vi "ziExample-HF2-RTK-PI.vi"() -> ()   [LabVIEW 2009]
doc: "This is an example for a Zurich Instruments HF2 instrument with RTK option installed. \nThis VI works together with a program for the real-time processor to implement two PI (Proportional-Integral) controllers. The controllers themselves run on the real-time processor. This VI communicates with the real-time processor to configure the controllers.\nThe program for the real-time processor is implemented in the file Main.c."
uses:
  <instrlib>/Zurich Instruments LabOne/Zurich Instruments LabOne.lvlib
panel:
  in  "pid2_invert":bool
  in  "pid1_invert":bool
  in  "pid2_input_select2":enum16{"X", "Y", "R", "Theta"}(ring) caption="Signal"
  in  "pid1_input_select2":enum16{"X", "Y", "R", "Theta"}(ring) caption="Signal"
  in  "pid2_max":sgl=1.0 format="%+7.3f"
  in  "pid2_min":sgl=-1.0 caption="Range" format="%+7.3f"
  in  "pid1_max":sgl=1.0 format="%+7.3f"
  in  "pid1_min":sgl=-1.0 caption="Range" format="%+7.3f"
  in  "pid2_output_select":enum16{"Aux 1", "Aux 2", "Aux 3", "Aux 4"}(ring)=enum."Aux 2" caption="Output"
  in  "pid1_output_select":enum16{"Aux 1", "Aux 2", "Aux 3", "Aux 4"}(ring) caption="Output"
  in  "stop":bool
  out "pid2_error":dbl caption="Error" format="%_5p"
  out "pid1_error":dbl caption="Error" format="%_5p"
  in  "Port":u16=8005
  in  "Host":string="localhost"
  in  "pid2_enable":bool caption="demodOn0"
  in  "pid1_enable":bool
  in  "pid2_set_point":sgl caption="Set point" format="%+7.3f"
  in  "pid2_tc_slider":sgl(slide)=1.0 scale=0.001..10.0 scale format="%#_6p"
  in  "pid2_kp_slider":sgl(slide)=0.001 scale=0.001..1.0 scale format="%#_6p"
  in  "pid2_input_select1":T1(ring)=enum."Demod 2" caption="Demodulator"
  in  "pid1_set_point":sgl caption="Set point" format="%+7.3f"
  in  "pid1_tc_slider":sgl(slide)=1.0 scale=0.001..10.0 scale format="%#_6p"
  in  "pid1_kp_slider":sgl(slide)=0.001 scale=0.001..1.0 scale format="%#_6p"
  in  "pid1_input_select1":T1(ring) caption="Demodulator"
  # "Prop. gain"
  # "Time constant (s)"
  # "En"
  # "Inv"
  # "Tested Devices:\n- HF2LI\n\nRequires the RTK \noption"
  # "PID1"
  # "to"
  # "Prop. gain"
  # "Time constant (s)"
  # "En"
  # "Inv"
  # "PID2"
  # "to"
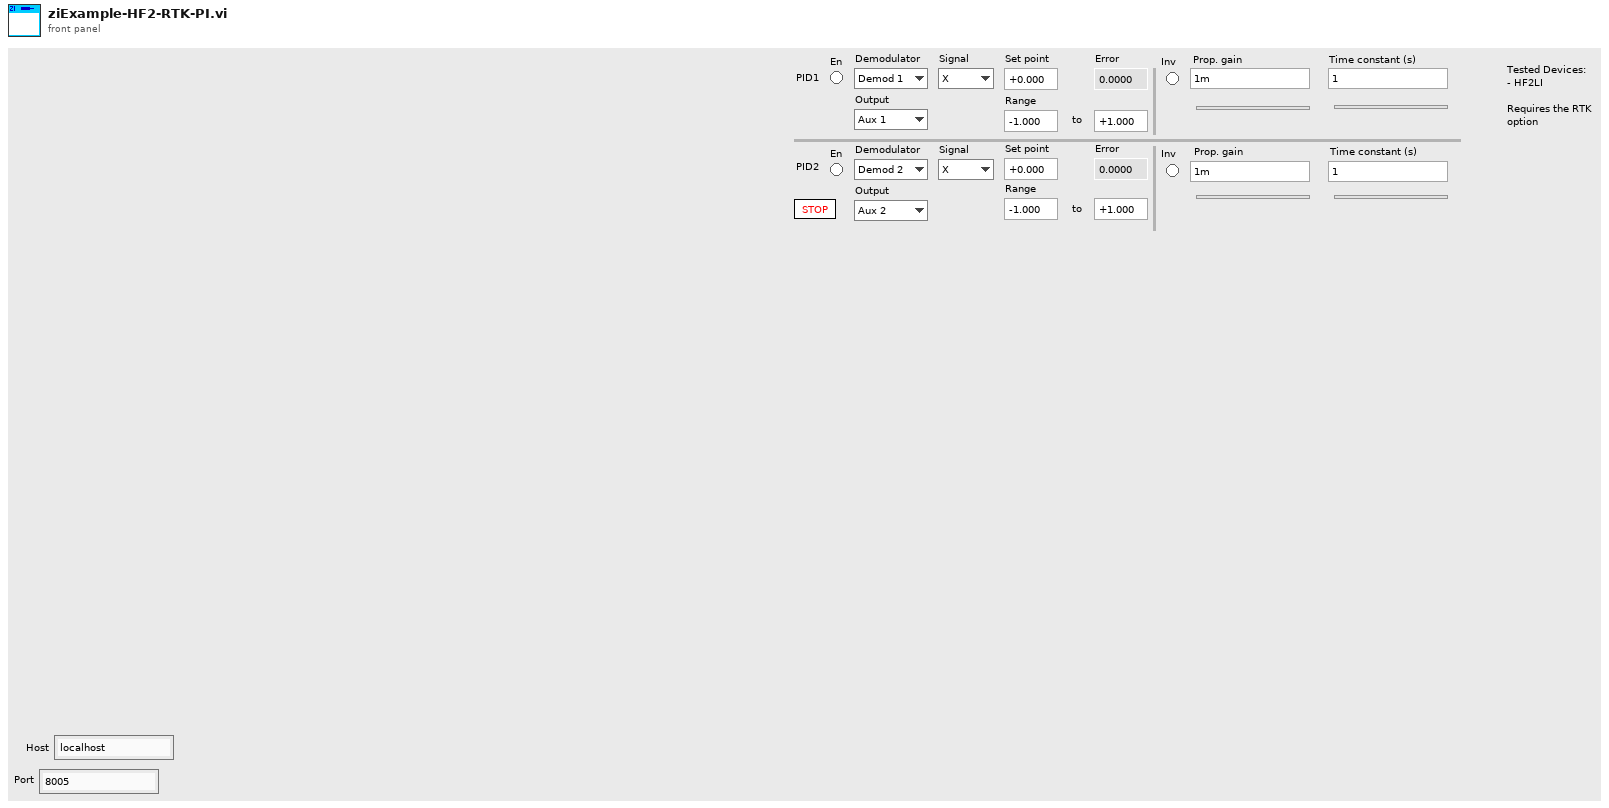
[diagram p1: front panel]
types:
  T1 = enum16{"Demod 1", "Demod 2", "Demod 3", "Demod 4", "Demod 5", "Demod 6", "Aux In 1", "Aux In 2"}
  T2 = typedef "Zurich Instruments LabOne.lvlib/ziTypeHandle.ctl" = cluster{"handleValid":bool, "Conn":u64, "Path Prefix":string, "Handle":u64, "Connected":bool, "Clockbase(s)":dbl}
  T3 = enum8{"Enabled", "Disabled", "Disabled and Grayed Out"}
  T4 = typedef "Zurich Instruments LabOne.lvlib/ziTypePollData.ctl" = cluster{"double":dbl, "Demod Sample":T5, "string":string, "Raw":u8[], "int":i32, "ScopeData":cluster{"wave":i16[], "dt (s)":dbl}, "DioInput":cluster{"Timestamp (ticks)":u64[], "Value":u32[]}, "AuxInput":cluster{"Timestamp (ticks)":u64[], "Val Ch0 (V)":dbl[], "Val Ch1 (V)":dbl[]}}
  T5 = typedef "Zurich Instruments LabOne.lvlib/ziTypeDemodSample.ctl" = cluster{"Channel":i32, "Timestamps (ticks)":u64[], "X (Vrms)":dbl[], "Y (Vrms)":dbl[], "Osc Phase (deg)":dbl[], "Freq (Hz)":dbl[], "DIO":u32[], "Aux In 0 (V)":dbl[], "Aux In 1 (V)":dbl[]}
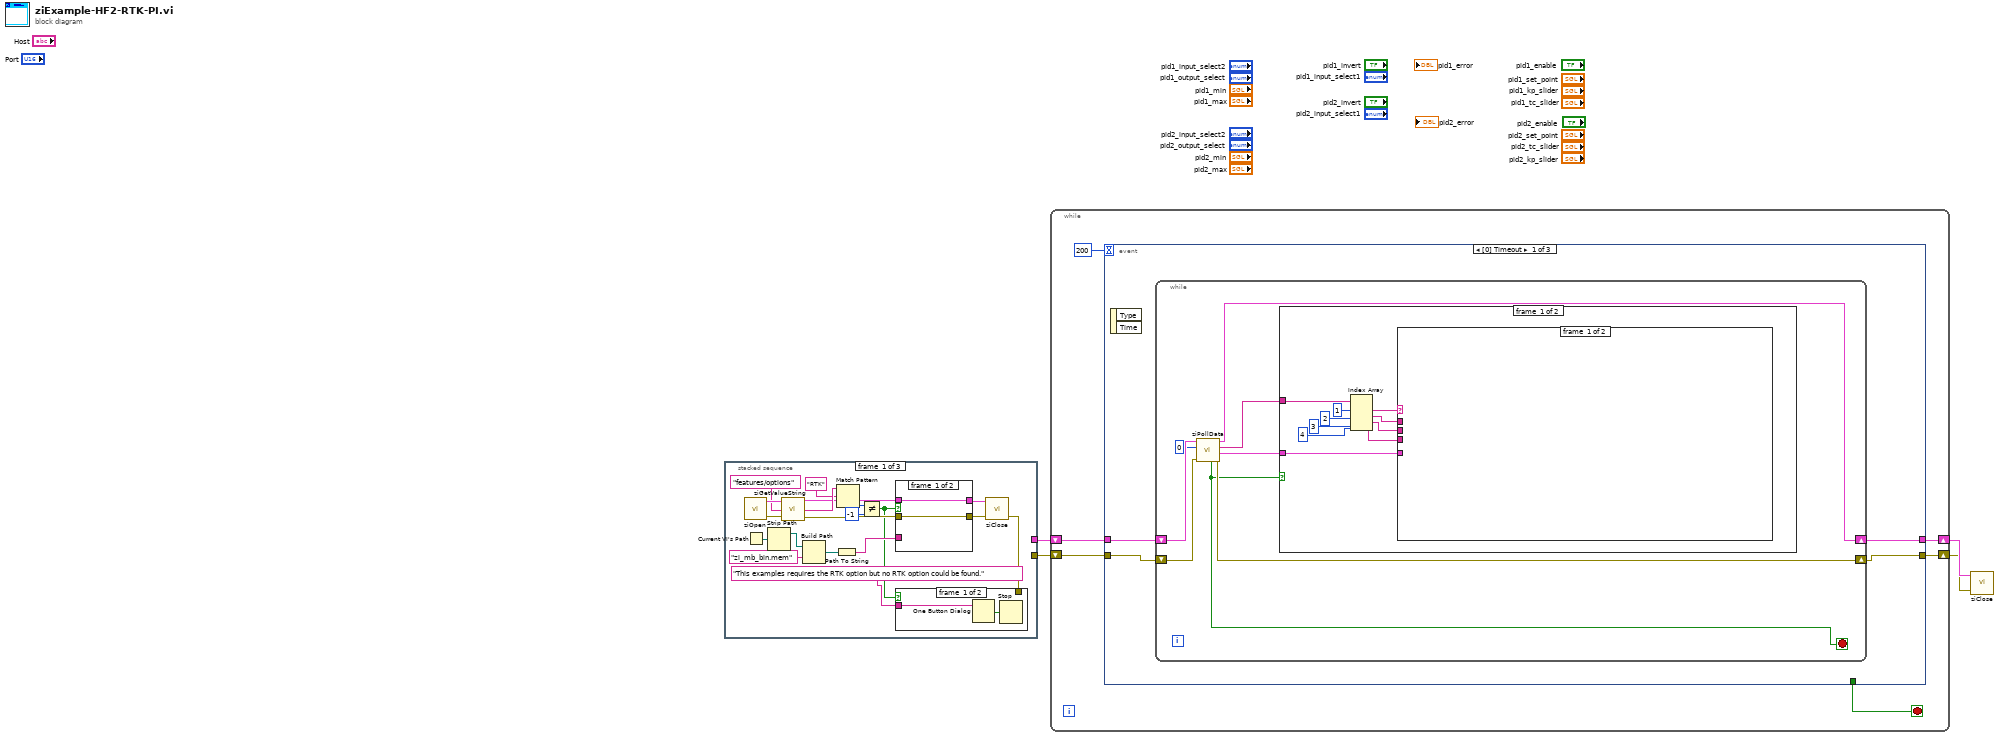
[diagram p0: block diagram]
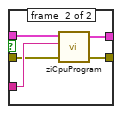
[diagram p3: hidden frame]
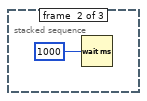
[diagram p4: hidden frame]
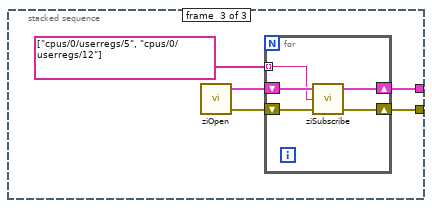
[diagram p5: hidden frame]
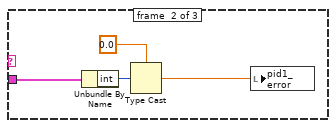
[diagram p9: hidden frame]
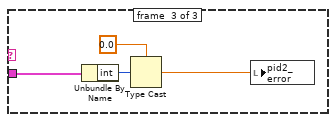
[diagram p10: hidden frame]
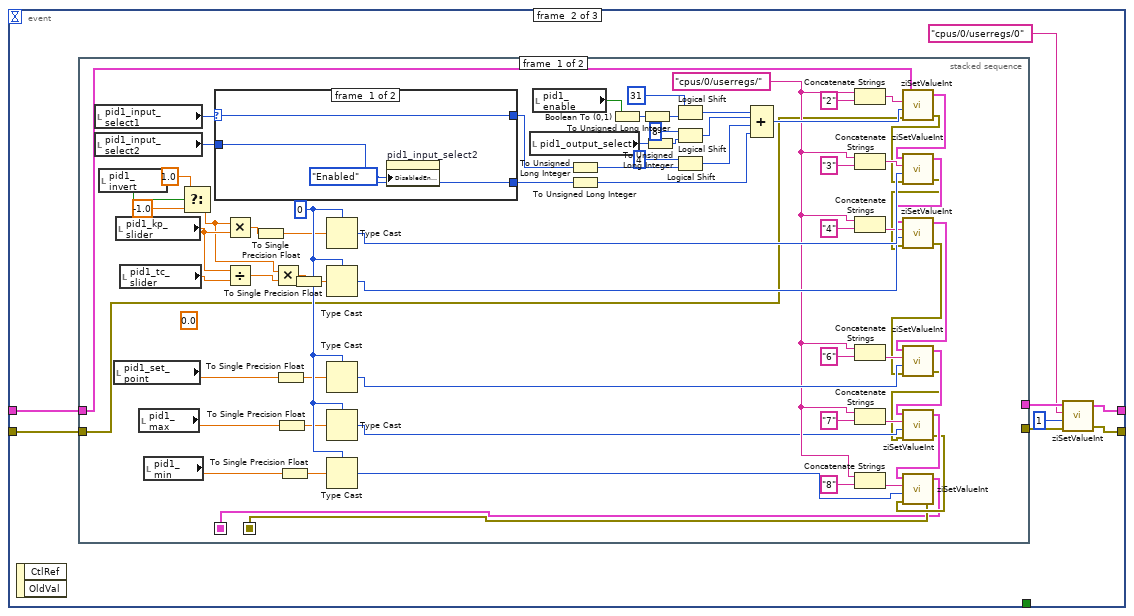
[diagram p12: hidden frame]
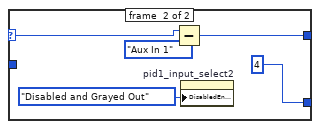
[diagram p13: hidden frame]
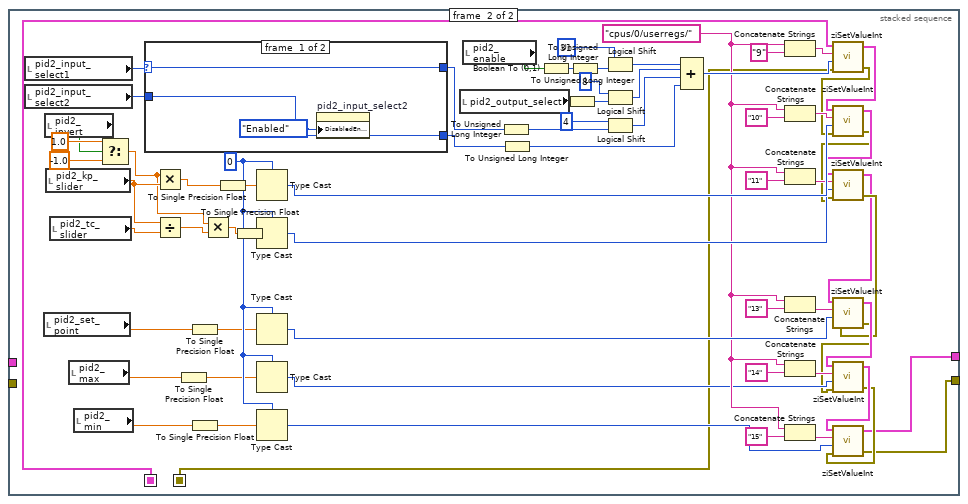
[diagram p14: hidden frame]
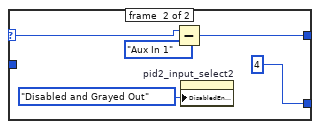
[diagram p15: hidden frame]
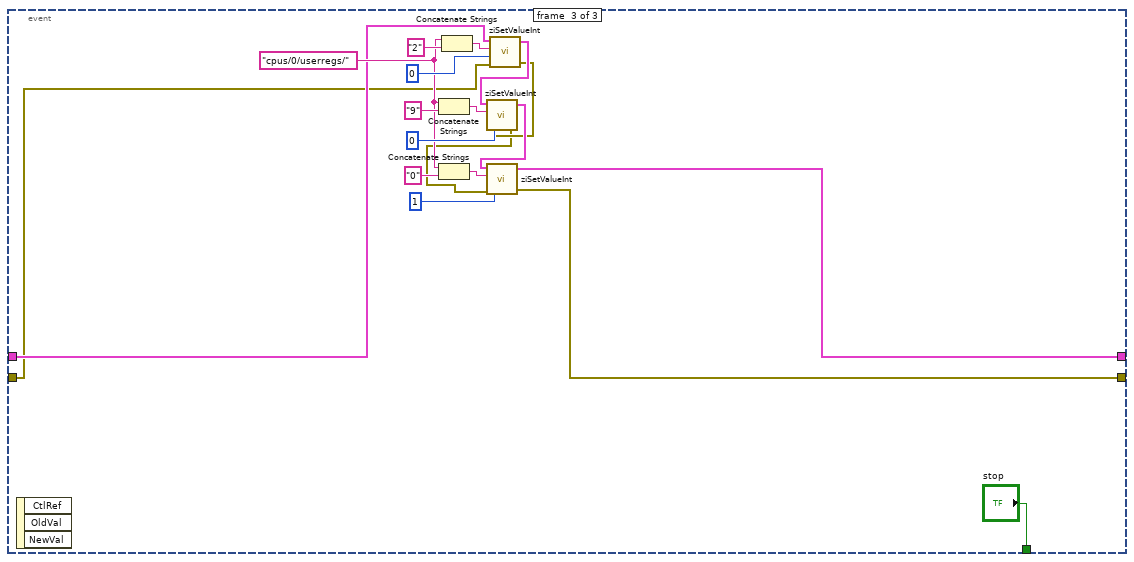
[diagram p16: hidden frame]
diagram:
  n1 = stacked-sequence {
    tunnel: [_ _ w37] -> w2
    tunnel: [_ _ w36] -> w1
    frame #0 {
      n2 = call <instrlib>:"ziOpen.vi"() -> ("Error Out"=w15:errorcluster, "HandleOut"=w16:T2)  [unwired: 4 in, 1 out]
      n3 = Current VI's Path() -> (path=w18:path)
      n4 = Strip Path(path=w18) -> (stripped path=w19:path)  [unwired: 1 out]
      n5 = call <instrlib>:"ziGetValueString.vi"("error in"=w15, "Path"="features/options", "Handle In"=w16) -> ("error out"=w9:errorcluster, "Value"=w13:string, "Handle Out"=w8:T2)
      n6 = Build Path(base path=w19, name or relative path="zi_mb_bin.mem") -> (appended path=w17:path)
      n7 = Path To String(path=w17) -> (string=w20:string)
      n8 = Match Pattern(string=w13, regular expression="RTK" ("Path")) -> (offset past match=w11:i32)  [unwired: 1 in, 3 out]
      n9 = Not Equal?(x=w11, y=-1) -> (x != y?=w7:bool)
      n10 = case shown="False" w7 {
        tunnel: [w26 w32] -> w22
        tunnel: [w27 w31] -> w21
        tunnel: w20 -> [_ w30]
        tunnel: w9 -> [w26 w29]
        tunnel: w8 -> [w27 w28]
        frame #0 {
        }
        frame #1 {
          n11 = call <instrlib>:"ziCpuProgram.vi"("error in"=w29, "Filename"=w30, "Handle In"=w28) -> ("error out"=w32:errorcluster, "Handle Out"=w31:T2)  [unwired: 2 in]
        }
      }
      n12 = call <instrlib>:"ziClose.vi"("Error In"=w22, "Handle In"=w21) -> ("Error Out"=w6:errorcluster)  [unwired: 3 out]
      n13 = case shown="False" w7 {
        tunnel: w6 -> [_ _]
        tunnel: "This examples requires the RTK option but no RTK option could be found." ("message") -> [w24 _]
        frame #0 {
          n14 = One Button Dialog(message=w24) -> (true=w25:bool)  [unwired: 1 in]
          n15 = Stop(stop? (T)=w25) -> ()
        }
        frame #1 {
        }
      }
    }
    frame #1 {
      n16 = Wait (ms)(milliseconds to wait=u32 1000) -> ()  [unwired: 1 out]
    }
    frame #2 {
      n17 = call <instrlib>:"ziOpen.vi"() -> ("Error Out"=w34:errorcluster, "HandleOut"=w35:T2)  [unwired: 4 in, 1 out]
      n18 = for {
        shift-right: [w41] -> w37
        shift-left: w35 -> [w43]
        shift-right: [w40] -> w36
        shift-left: w34 -> [w42]
        tunnel: string[] ["cpus/0/userregs/5", "cpus/0/userregs/12"] -> [w39] mode=indexing
        n19 = call <instrlib>:"ziSubscribe.vi"("error in"=w42, "Path ()"=w39, "Handle In"=w43) -> ("error out"=w40:errorcluster, "Handle Out"=w41:T2)  [unwired: 1 in]
      }
    }
  }
  n20 = while {
    shift-right: [w47] -> w4
    shift-left: w2 -> [w49]
    shift-right: [w46] -> w3
    shift-left: w1 -> [w48]
    stop <- w45 stop-if-true
    n21 = event shown="[0] Timeout" {
      selector: _ -> [_ _ _]
      dyn-events: _ -> [_ _ _]
      timeout: 200 -> [_ _ _]
      tunnel: w49 -> [w53 w96 w256]
      tunnel: w48 -> [w52 w95 w252]
      tunnel: [w51 w93 w255] -> w47
      tunnel: [w50 w94 w249] -> w46
      tunnel: [_ _ "stop"] -> w45
      event #0 {
        n22 = event-data() -> ()  [unwired: 3 out]
        n23 = while {
          shift-right: [w59] -> w51
          shift-left: w53 -> [w61]
          shift-right: [w58] -> w50
          shift-left: w52 -> [w60]
          stop <- w57 stop-if-true
          n24 = call <instrlib>:"ziPollData.vi"("Error In"=w60, "TimeOut ms (50)"=0, "Handle In"=w61) -> ("Error Out"=w58:errorcluster, "Data Out"=w55:T4, "PathArray"=w56:string[], "Handle Out"=w59:T2, "Timed Out"=w57:bool)  [unwired: 3 in, 1 out]
          n25 = case shown="False" w57 {
            tunnel: w56 -> [w71 _]
            tunnel: w55 -> [w66 _]
            frame #0 {
              n26 = Index Array(array=w71, index #1=1 ("index"), index #2=2 ("index"), index #3=3 ("index"), index #4=4 ("index")) -> (element #1=w69:string, element #2=w67:string, element #3=w64:string, element #4=w62:string)
              n27 = case shown="\"CPUS\"" w69 {
                tunnel: w67 -> [_ w75]
                tunnel: w66 -> [_ w73]
                tunnel: w64 -> [_ w74]
                tunnel: w62 -> [_ w72]
                frame #0 {
                }
                frame #1 {
                  n28 = case shown="\"0\"" w75 {
                    tunnel: w74 -> [_ w78]
                    tunnel: w73 -> [_ w77]
                    tunnel: w72 -> [_ w76]
                    frame #0 {
                    }
                    frame #1 {
                      n29 = case shown="\"USERREGS\"" w78 {
                        tunnel: w77 -> [_ w79]
                        tunnel: w76 -> [_ w80]
                        frame #0 {
                        }
                        frame #1 {
                          n30 = case shown="\"5\"" w80 {
                            tunnel: w79 -> [_ w84 w88]
                            frame #0 {
                            }
                            frame #1 {
                              n31 = Unbundle By Name(w84) -> ("int"=w83:i32)
                              n32 = Type Cast(type=sgl 0.0, x=w83) -> (*(type *) &x=w81:sgl)
                              n33 = local write "pid1_error"(w81) -> ()
                            }
                            frame #2 {
                              n34 = Unbundle By Name(w88) -> ("int"=w87:i32)
                              n35 = Type Cast(type=sgl 0.0, x=w87) -> (*(type *) &x=w85:sgl)
                              n36 = local write "pid2_error"(w85) -> ()
                            }
                          }
                        }
                      }
                    }
                  }
                }
              }
            }
            frame #1 {
            }
          }
        }
      }
      event #1 {
        n37 = event-data() -> ()  [unwired: 3 out]
        n38 = stacked-sequence {
          seq-local: [w115 _] -> [_ w193]
          seq-local: [w116 _] -> [_ w192]
          tunnel: w96 -> [w126 _]
          tunnel: w95 -> [w125 _]
          tunnel: [_ w195] -> w91
          tunnel: [_ w194] -> w92
          frame #0 {
            w136 = 0
            w129 = "cpus/0/userregs/"
            (unwired) sgl 0.0 ("number")
            n39 = local read "pid1_input_select1"() -> (w162:T1)
            n40 = local read "pid1_input_select2"() -> (w161:enum16{"X", "Y", "R", "Theta"})
            n41 = local read "pid1_invert"() -> (w106:bool)
            n42 = local read "pid1_set_point"() -> (w140:sgl)
            n43 = local read "pid1_kp_slider"() -> (w164:sgl)
            n44 = local read "pid1_tc_slider"() -> (w163:sgl)
            n45 = local read "pid1_max"() -> (w135:sgl)
            n46 = local read "pid1_min"() -> (w134:sgl)
            n47 = Select(t=1.0, s=w106, f=-1.0) -> (s? t:f=w102:dbl)
            n48 = case shown="\"Aux In 1\", \"Aux In 2\"" w162 {
              selector: w162 -> [w167 w172]
              tunnel: [w167 w170] -> w154
              tunnel: [w166 4] -> w153
              tunnel: w161 -> [w166 _]
              frame #0 {
                n49 = property on="pid1_input_select2" class="Enum (strict)"("DisabledEnum"=T3."Enabled" ("Disabled")) -> ()  [unwired: 2 in, 2 out]
              }
              frame #1 {
                n50 = Subtract(x=w172, y=T1."Aux In 1") -> (x-y=w170:u16)
                n51 = property on="pid1_input_select2" class="Enum (strict)"("DisabledEnum"=T3."Disabled and Grayed Out" ("Disabled")) -> ()  [unwired: 2 in, 2 out]
              }
            }
            n52 = Multiply(x=w102, y=w164) -> (x*y=w146:dbl)
            n53 = Divide(x=w164, y=w163) -> (x/y=w103:sgl)
            n54 = To Single Precision Float(number=w146) -> (single precision float=w101:sgl)
            n55 = Multiply(x=w102, y=w103) -> (x*y=w144:dbl)
            n56 = To Single Precision Float(number=w140) -> (single precision float=w99:sgl)
            n57 = To Single Precision Float(number=w135) -> (single precision float=w98:sgl)
            n58 = To Single Precision Float(number=w134) -> (single precision float=w97:sgl)
            n59 = To Single Precision Float(number=w144) -> (single precision float=w100:sgl)
            n60 = Type Cast(type=w136, x=w101) -> (*(type *) &x=w145:i32)
            n61 = Type Cast(type=w136, x=w100) -> (*(type *) &x=w141:i32)
            n62 = Type Cast(type=w136, x=w99) -> (*(type *) &x=w137:i32)
            n63 = Type Cast(type=w136, x=w98) -> (*(type *) &x=w127:i32)
            n64 = Type Cast(type=w136, x=w97) -> (*(type *) &x=w128:i32)
            n65 = local read "pid1_output_select"() -> (w149:enum16{"Aux 1", "Aux 2", "Aux 3", "Aux 4"})
            n66 = local read "pid1_enable"() -> (w160:bool)
            n67 = To Unsigned Long Integer(number=w154) -> (unsigned 32bit integer=w113:u32)
            n68 = To Unsigned Long Integer(number=w153) -> (unsigned 32bit integer=w110:u32)
            n69 = Boolean To (0,1)(Boolean=w160) -> (0, 1=w158:i16)
            n70 = To Unsigned Long Integer(number=w158) -> (unsigned 32bit integer=w114:u32)
            n71 = To Unsigned Long Integer(number=w149) -> (unsigned 32bit integer=w112:u32)
            n72 = Logical Shift(y=u32 31, x=w114) -> (x << y=w156:u32)
            n73 = Logical Shift(y=u32 8, x=w112) -> (x << y=w111:u32)
            n74 = Logical Shift(y=u32 4, x=w113) -> (x << y=w109:u32)
            n75 = Compound Arithmetic op=ADD(w156, w111, w109, w110) -> (w159:u32)
            n76 = Concatenate Strings(w129, "2" ("string")) -> (w152:string)
            n77 = Concatenate Strings(w129, "3" ("string")) -> (w148:string)
            n78 = Concatenate Strings(w129, "4" ("string")) -> (w143:string)
            n79 = Concatenate Strings(w129, "6" ("string")) -> (w139:string)
            n80 = Concatenate Strings(w129, "7" ("string")) -> (w132:string)
            n81 = Concatenate Strings(w129, "8" ("string")) -> (w131:string)
            n82 = call <instrlib>:"ziSetValueInt.vi"("Error in"=w125, "Value"=w159, "Path"=w152, "Handle in"=w126) -> ("Error out"=w120:errorcluster, "Handle out"=w124:T2)  [unwired: 1 in]
            n83 = call <instrlib>:"ziSetValueInt.vi"("Error in"=w120, "Value"=w145, "Path"=w148, "Handle in"=w124) -> ("Error out"=w119:errorcluster, "Handle out"=w123:T2)  [unwired: 1 in]
            n84 = call <instrlib>:"ziSetValueInt.vi"("Error in"=w119, "Value"=w141, "Path"=w143, "Handle in"=w123) -> ("Error out"=w108:errorcluster, "Handle out"=w107:T2)  [unwired: 1 in]
            n85 = call <instrlib>:"ziSetValueInt.vi"("Error in"=w108, "Value"=w137, "Path"=w139, "Handle in"=w107) -> ("Error out"=w118:errorcluster, "Handle out"=w122:T2)  [unwired: 1 in]
            n86 = call <instrlib>:"ziSetValueInt.vi"("Error in"=w118, "Value"=w127, "Path"=w132, "Handle in"=w122) -> ("Error out"=w117:errorcluster, "Handle out"=w121:T2)  [unwired: 1 in]
            n87 = call <instrlib>:"ziSetValueInt.vi"("Error in"=w117, "Value"=w128, "Path"=w131, "Handle in"=w121) -> ("Error out"=w116:errorcluster, "Handle out"=w115:T2)  [unwired: 1 in]
          }
          frame #1 {
            w213 = 0
            w206 = "cpus/0/userregs/"
            n88 = local read "pid2_input_select1"() -> (w238:T1)
            n89 = local read "pid2_input_select2"() -> (w237:enum16{"X", "Y", "R", "Theta"})
            n90 = local read "pid2_set_point"() -> (w217:sgl)
            n91 = local read "pid2_invert"() -> (w178:bool)
            n92 = local read "pid2_kp_slider"() -> (w240:sgl)
            n93 = local read "pid2_tc_slider"() -> (w239:sgl)
            n94 = local read "pid2_max"() -> (w212:sgl)
            n95 = local read "pid2_min"() -> (w211:sgl)
            n96 = Select(t=1.0, s=w178, f=-1.0) -> (s? t:f=w181:dbl)
            n97 = case shown="\"Aux In 1\", \"Aux In 2\"" w238 {
              selector: w238 -> [w243 w248]
              tunnel: [w243 w246] -> w230
              tunnel: [w242 4] -> w188
              tunnel: w237 -> [w242 _]
              frame #0 {
                n98 = property on="pid2_input_select2" class="Enum (strict)"("DisabledEnum"=T3."Enabled" ("Disabled")) -> ()  [unwired: 2 in, 2 out]
              }
              frame #1 {
                n99 = Subtract(x=w248, y=T1."Aux In 1") -> (x-y=w246:u16)
                n100 = property on="pid2_input_select2" class="Enum (strict)"("DisabledEnum"=T3."Disabled and Grayed Out" ("Disabled")) -> ()  [unwired: 2 in, 2 out]
              }
            }
            n101 = Multiply(x=w181, y=w240) -> (x*y=w223:dbl)
            n102 = Divide(x=w240, y=w239) -> (x/y=w182:sgl)
            n103 = To Single Precision Float(number=w212) -> (single precision float=w174:sgl)
            n104 = To Single Precision Float(number=w217) -> (single precision float=w175:sgl)
            n105 = To Single Precision Float(number=w211) -> (single precision float=w173:sgl)
            n106 = Multiply(x=w181, y=w182) -> (x*y=w221:dbl)
            n107 = To Single Precision Float(number=w223) -> (single precision float=w177:sgl)
            n108 = To Single Precision Float(number=w221) -> (single precision float=w176:sgl)
            n109 = Type Cast(type=w213, x=w177) -> (*(type *) &x=w222:i32)
            n110 = Type Cast(type=w213, x=w176) -> (*(type *) &x=w218:i32)
            n111 = Type Cast(type=w213, x=w175) -> (*(type *) &x=w214:i32)
            n112 = Type Cast(type=w213, x=w174) -> (*(type *) &x=w204:i32)
            n113 = Type Cast(type=w213, x=w173) -> (*(type *) &x=w205:i32)
            n114 = local read "pid2_output_select"() -> (w226:enum16{"Aux 1", "Aux 2", "Aux 3", "Aux 4"})
            n115 = local read "pid2_enable"() -> (w236:bool)
            n116 = To Unsigned Long Integer(number=w230) -> (unsigned 32bit integer=w186:u32)
            n117 = To Unsigned Long Integer(number=w188) -> (unsigned 32bit integer=w185:u32)
            n118 = Boolean To (0,1)(Boolean=w236) -> (0, 1=w234:i16)
            n119 = To Unsigned Long Integer(number=w226) -> (unsigned 32bit integer=w190:u32)
            n120 = To Unsigned Long Integer(number=w234) -> (unsigned 32bit integer=w191:u32)
            n121 = Logical Shift(y=i8 31, x=w191) -> (x << y=w232:u32)
            n122 = Logical Shift(y=i16 8, x=w190) -> (x << y=w189:u32)
            n123 = Logical Shift(y=i16 4, x=w186) -> (x << y=w187:u32)
            n124 = Compound Arithmetic op=ADD(w232, w189, w187, w185) -> (w235:u32)
            n125 = Concatenate Strings(w206, "9" ("string")) -> (w229:string)
            n126 = Concatenate Strings(w206, "10" ("string")) -> (w225:string)
            n127 = Concatenate Strings(w206, "11" ("string")) -> (w220:string)
            n128 = Concatenate Strings(w206, "13" ("string")) -> (w216:string)
            n129 = Concatenate Strings(w206, "14" ("string")) -> (w209:string)
            n130 = Concatenate Strings(w206, "15" ("string")) -> (w208:string)
            n131 = call <instrlib>:"ziSetValueInt.vi"("Error in"=w192, "Value"=w235, "Path"=w229, "Handle in"=w193) -> ("Error out"=w199:errorcluster, "Handle out"=w203:T2)  [unwired: 1 in]
            n132 = call <instrlib>:"ziSetValueInt.vi"("Error in"=w199, "Value"=w222, "Path"=w225, "Handle in"=w203) -> ("Error out"=w198:errorcluster, "Handle out"=w202:T2)  [unwired: 1 in]
            n133 = call <instrlib>:"ziSetValueInt.vi"("Error in"=w198, "Value"=w218, "Path"=w220, "Handle in"=w202) -> ("Error out"=w184:errorcluster, "Handle out"=w183:T2)  [unwired: 1 in]
            n134 = call <instrlib>:"ziSetValueInt.vi"("Error in"=w184, "Value"=w214, "Path"=w216, "Handle in"=w183) -> ("Error out"=w197:errorcluster, "Handle out"=w201:T2)  [unwired: 1 in]
            n135 = call <instrlib>:"ziSetValueInt.vi"("Error in"=w197, "Value"=w204, "Path"=w209, "Handle in"=w201) -> ("Error out"=w196:errorcluster, "Handle out"=w200:T2)  [unwired: 1 in]
            n136 = call <instrlib>:"ziSetValueInt.vi"("Error in"=w196, "Value"=w205, "Path"=w208, "Handle in"=w200) -> ("Error out"=w194:errorcluster, "Handle out"=w195:T2)  [unwired: 1 in]
          }
        }
        n137 = call <instrlib>:"ziSetValueInt.vi"("Error in"=w92, "Value"=i64 1, "Path"="cpus/0/userregs/0", "Handle in"=w91) -> ("Error out"=w94:errorcluster, "Handle out"=w93:T2)  [unwired: 1 in]
      }
      event #2 {
        w258 = "cpus/0/userregs/"
        n138 = event-data() -> ()  [unwired: 4 out]
        n139 = Concatenate Strings(w258, "9" ("string")) -> (w264:string)
        n140 = Concatenate Strings(w258, "0" ("string")) -> (w260:string)
        n141 = Concatenate Strings(w258, "2" ("string")) -> (w265:string)
        n142 = call <instrlib>:"ziSetValueInt.vi"("Error in"=w252, "Value"=i64 0, "Path"=w265, "Handle in"=w256) -> ("Error out"=w251:errorcluster, "Handle out"=w253:T2)  [unwired: 1 in]
        n143 = call <instrlib>:"ziSetValueInt.vi"("Error in"=w251, "Value"=i64 0, "Path"=w264, "Handle in"=w253) -> ("Error out"=w250:errorcluster, "Handle out"=w254:T2)  [unwired: 1 in]
        n144 = call <instrlib>:"ziSetValueInt.vi"("Error in"=w250, "Value"=i64 1, "Path"=w260, "Handle in"=w254) -> ("Error out"=w249:errorcluster, "Handle out"=w255:T2)  [unwired: 1 in]
      }
    }
  }
  n145 = call <instrlib>:"ziClose.vi"("Error In"=w3, "Handle In"=w4) -> ()  [unwired: 4 out]
